vi "MT Generate ASK Symbol Map.vi"(0 "symbol values":i32[](array[numeric]), 11 "error in (no error)":errorcluster) -> (4 "symbol map":cdb[](array[numeric]) format="%.3f", 6 "bits per symbol":i32, 15 "error out":errorcluster)   [LabVIEW 2020, in "niDMT.lvlib"]
uses:
  <vilib>/addons/Modulation/niDMT.lvlib
  <vilib>/addons/Modulation/niAMT.lvlib
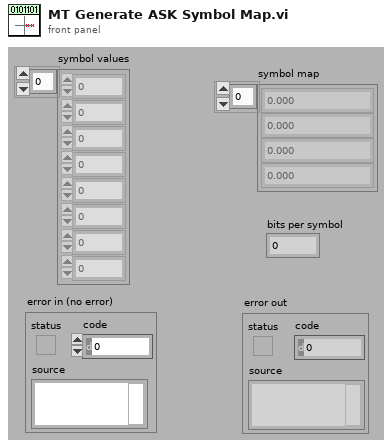
[diagram p1: front panel]
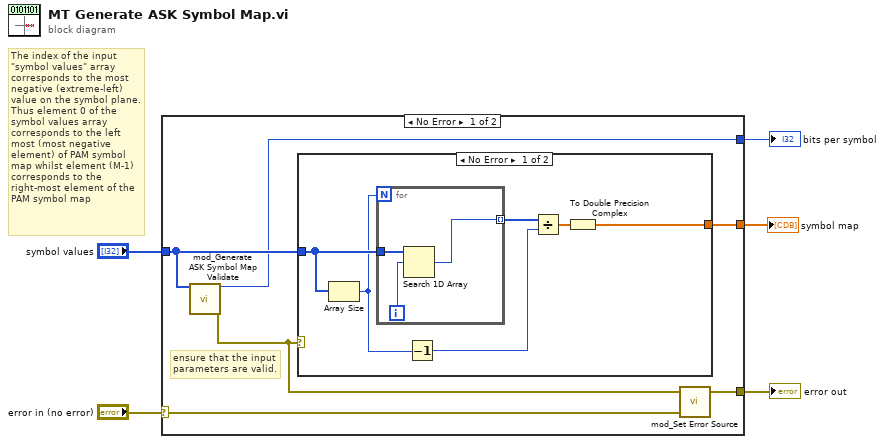
[diagram p0: block diagram]
diagram:
  # "The index of the input \"symbol values\" array \ncorresponds to the most \nnegative (extreme-left) \nvalue on the symbol plane.\nThus element 0 of the \nsymbol values array corresponds to the left most (most negative element) of PAM symbol map whilst element (M-1)\ncorresponds to the right-most element of the PAM symbol map"
  n1 = case shown="No Error" "error in (no error)" {
    selector: "error in (no error)" -> [w11 w21]
    tunnel: "symbol values" -> [w9 _]
    tunnel: [w10 w21] -> w4
    tunnel: [w7 _] -> w2
    tunnel: [w6 _] -> w1
    frame No Error {
      # "ensure that the input parameters are valid."
      n2 = call <vilib>:"mod_Generate ASK Symbol Map Validate.vi"("Symbol Map"=w9) -> ("bits per symbol"=w7:i32, "error out"=w8:errorcluster)  [unwired: 13 out]
      n3 = case shown="No Error" w8 {
        tunnel: w9 -> [w17 _]
        tunnel: [w12 _] -> w6
        frame No Error {
          n4 = Array Size(array=w17) -> (size(s)=w15:i32)
          n5 = for {
            N: w15 -> [_]
            tunnel: w17 -> [w20]
            tunnel: [w18] -> w16 mode=indexing
            i -> [w19]
            n6 = Search 1D Array(1D array=w20, element=w19) -> (index of element=w18:i32)  [unwired: 1 out]
          }
          n7 = Decrement(x=w15) -> (x-1=w14:i32)
          n8 = Divide(x=w16, y=w14) -> (x/y=w13:dbl[])
          n9 = To Double Precision Complex(1:w13) -> (0:w12:cdb[])
        }
        frame Error {
        }
      }
      n10 = call <vilib>:"mod_Set Error Source.vi"("initial error in (no error)"=w11, "final error in (no error)"=w8) -> ("error out"=w10:errorcluster)  [unwired: 3 out]
    }
    frame Error {
    }
  }
  "error out" <- w4
  "symbol map" <- w1
  "bits per symbol" <- w2
